vi "pop_dialog_if_no_duplicate.vi"(1 "FirstTime":bool, 2 "State In in":T1 {"BlockNodeState"."Draw Style" items=["FunctionBlock", "ExpressVI", "Variable", "Elemental I/O", "32x32 Icon", "FunctionBlockCompact"]; "BlockNodeState"."Terminal Data"."Terminal Flags" format="%.0b"}) -> (8 "NeedUpdate":bool, 9 "State In out":T1 {"BlockNodeState"."Draw Style" items=["FunctionBlock", "ExpressVI", "Variable", "Elemental I/O", "32x32 Icon", "FunctionBlockCompact"]; "BlockNodeState"."Terminal Data"."Terminal Flags" format="%.0b"})   [LabVIEW 2018]
uses:
  State.ctl
  <vilib>/BlockNodeSupport/BlockNodeState.ctl
  <vilib>/BlockNodeSupport/TerminalData.ctl
  <vilib>/picture/picture.llb/imagedata.ctl
  command_spec.ctl
  N9010A_SCPI Node.xnode
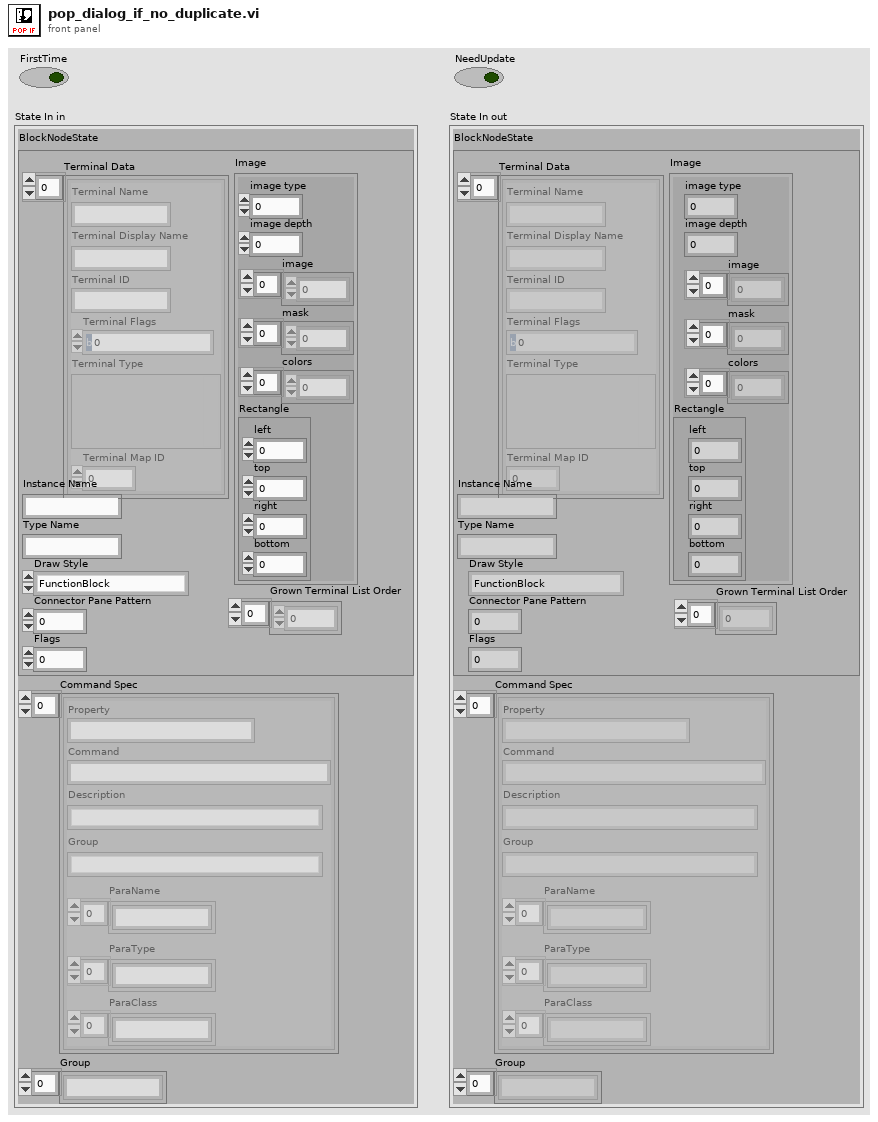
[diagram p1: front panel]
types:
  T1 = typedef "N9010A_SCPI Node.xnode/State.ctl" = cluster{"BlockNodeState":T2, "Command Spec":T5, "Group":string[]}
  T2 = typedef "BlockNodeState.ctl" = cluster{"Terminal Data":T3[], "Instance Name":string, "Type Name":string, "Draw Style":i32, "Connector Pane Pattern":i32, "Flags":i32, "Grown Terminal List Order":i32[], "Image":T4}
  T3 = typedef "TerminalData.ctl" = cluster{"Terminal Name":string, "Terminal Display Name":string, "Terminal ID":string, "Terminal Flags":i32, "Terminal Type":variant, "Terminal Map ID":i32}
  T4 = typedef "imagedata.ctl" = cluster{"image type":i32, "image depth":i32, "image":u8[], "mask":u8[], "colors":u32[], "Rectangle":cluster{"left":i16, "top":i16, "right":i16, "bottom":i16}}
  T5 = typedef "command_spec.ctl" = cluster{"Property":string, "Command":string, "Description":string, "Group":string, "ParaName":string[], "ParaType":string[], "ParaClass":string[]}[]
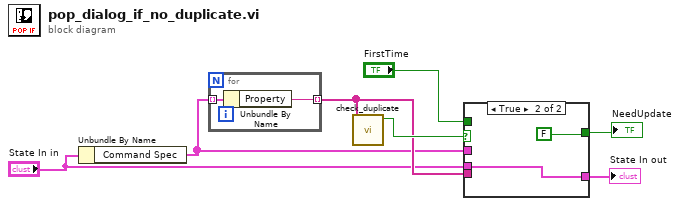
[diagram p0: block diagram]
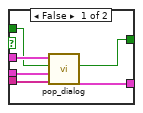
[diagram p2: hidden frame]
diagram:
  n1 = Unbundle By Name("State In in") -> ("Command Spec"=w4:T5)
  n2 = for {
    tunnel: w4 -> [w9] mode=indexing
    tunnel: [w8] -> w5 mode=indexing
    n3 = Unbundle By Name(w9) -> ("Property"=w8:string)
  }
  n4 = call "check_duplicate.vi"("Array"=w5) -> ("hasDuplicate"=w6:bool)  [unwired: 10 in]
  n5 = case shown="True" w6 {
    tunnel: [w15 w17] -> w1
    tunnel: [w14 FALSE] -> w2
    tunnel: "State In in" -> [w13 w17]
    tunnel: w4 -> [w12 _]
    tunnel: w5 -> [w11 _]
    tunnel: "FirstTime" -> [w10 _]
    frame False {
      n6 = call "pop_dialog.vi"("Property"=w11, "State In"=w13, "FirstTime"=w10, "Command Spec"=w12) -> ("State Out"=w15:T1, "NeedUpdate"=w14:bool)  [unwired: 6 in]
    }
    frame True {
    }
  }
  "NeedUpdate" <- w2
  "State In out" <- w1
